vi "HHMI - Count U16.vi"(7 "Reset?":bool, 10 "Increment?":bool) -> (2 "total # counted\n(Reset occurs \nprior to Increment)":u16)   [LabVIEW 2013]
doc: "Counts up. Reset returns count to zero. Increment occurs after Reset."
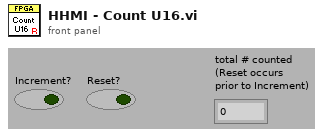
[diagram p1: front panel]
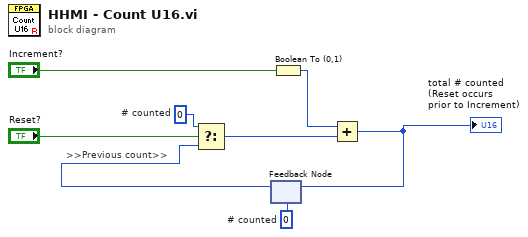
[diagram p0: block diagram]
diagram:
  w5 = u16 0  # # counted
  w8 = u16 0  # # counted
  # ">>Previous count>>"
  n1 = feedback #1(w8) -> (w6:u16)
  n2 = Select(t=w5, s="Reset?", f=w6) -> (s? t:f=w3:u16)
  n3 = Boolean To (0,1)(Boolean="Increment?") -> (0, 1=w1:i16)
  n4 = Add(x=w1, y=w3) -> (x+y=w2:u16)
  "total # counted\n(Reset occurs \nprior to Increment)" <- w2
  n5 = feedback-in #1(w2) -> ()
